vi "Parse Parameter.vi"(6 "error text in":string, 7 "direction":T1, 8 "error in":errorcluster, 11 "node in":refnum<k20>) -> (0 "error out":errorcluster, 3 "parametesrs":T2[](array[typedef]))   [LabVIEW 2023, in "ARINC 429 Import.lvlib"]
uses:
  ARINC 429 Import.lvlib
  <vilib>/NI/NI VeriStand Encoding and Decoding/Encoding.ctl
  Read Tag Element (String).vi
  Read Tag Element (DBL).vi
  Read Tag Element (I32).vi
  Shared/Parameter Definition.ctl
  Shared/VS Channel Definition for Parameter.ctl
  Read Tag Element (Boolean).vi
  Shared/Direction.ctl
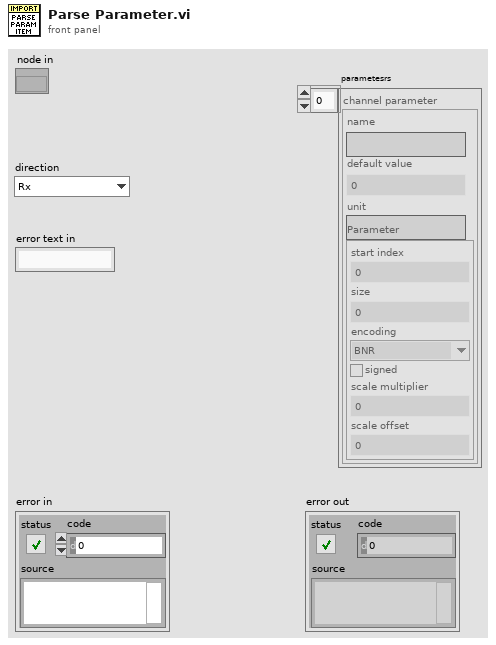
[diagram p1: front panel]
types:
  T1 = typedef "Direction.ctl" = enum16{"Rx", "Tx"}
  T2 = typedef "VS Channel Definition for Parameter.ctl" = cluster{"name":string, "default value":dbl, "unit":string, "Parameter":T3}
  T3 = typedef "Parameter Definition.ctl" = cluster{"start index":i32, "size":i32, "encoding":T4, "signed":bool, "scale multiplier":dbl, "scale offset":dbl}
  T4 = typedef "Encoding and Decoding.lvlib/Encoding.ctl" = enum16{"BNR", "BCD", "Discrete"}
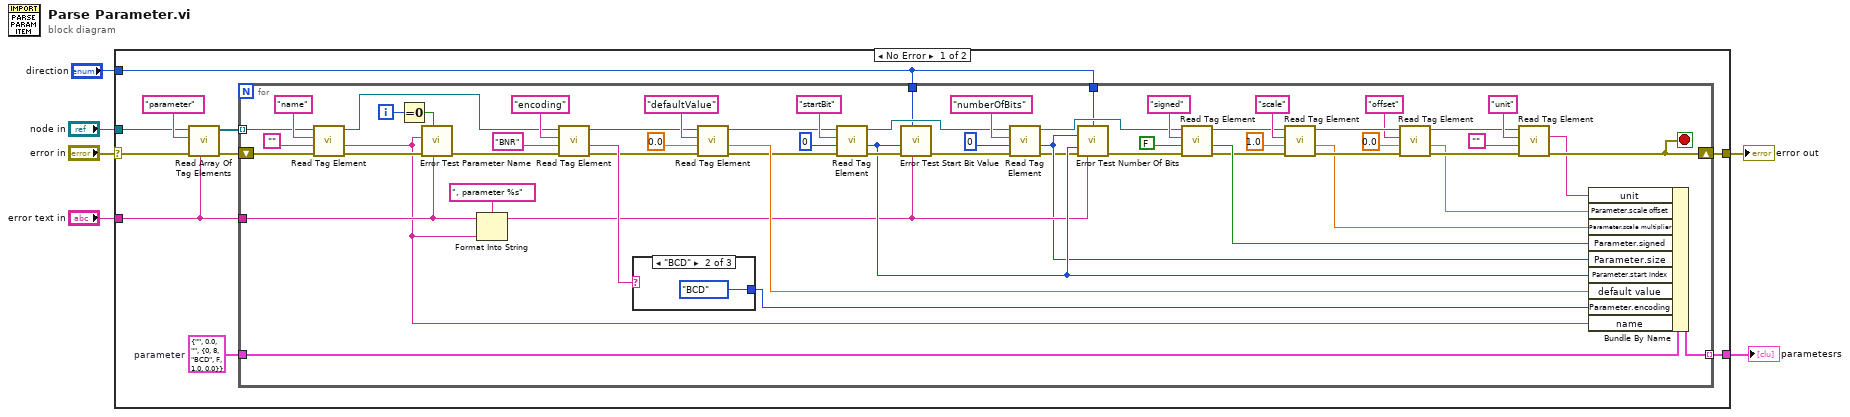
[diagram p0: block diagram]
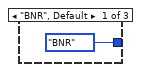
[diagram p2: hidden frame]
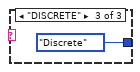
[diagram p3: hidden frame]
diagram:
  n1 = case shown="No Error" "error in" {
    selector: "error in" -> [w11 w79]
    tunnel: "node in" -> [w13 _]
    tunnel: [w12 w79] -> w5
    tunnel: "error text in" -> [w10 _]
    tunnel: [w9 _] -> w2
    tunnel: "direction" -> [w7 _]
    frame No Error {
      w8 = T2 {"name"="", "default value"=0.0, "unit"="", "Parameter"={"start index"=0, "size"=8, "encoding"=enum."BCD", "signed"=FALSE, "scale multiplier"=1.0, "scale offset"=0.0}}  # parameter
      n2 = call "Read Array Of Tag Elements.vi"("error text in"=w10, "error in"=w11, "tag name"="parameter" ("Tag Name"), "node in"=w13) -> ("error out"=w15:errorcluster, "array of elements"=w14:refnum<k20>[])  [unwired: 6 in]
      n3 = for {
        shift-right: [w38] -> w12
        shift-left: w15 -> [w73]
        tunnel: w14 -> [w41] mode=indexing
        tunnel: w10 -> [w31]
        tunnel: [w25] -> w9 mode=indexing
        tunnel: w8 -> [w24]
        tunnel: w7 -> [w23]
        tunnel: w7 -> [w20]
        i -> [w34]
        stop <- w38 stop-if-true
        n4 = call-poly "Read Tag Element.vi"("error in"=w73, "default"="", "Tag Name"="name", "node in"=w41) -> ("error out"=w36:errorcluster, "value"=w29:string, "node out"=w32:refnum<k20>)  [unwired: 5 in]
        n5 = Equal To 0?(x=w34) -> (x = 0?=w33:bool)
        n6 = call "Error Test Parameter Name.vi"("error text in"=w31, "reset (F)"=w33, "error in"=w36, "parameter name"=w29) -> ("error out"=w35:errorcluster)  [unwired: 7 in]
        n7 = Format Into String(format string=", parameter %s", initial string=w31, w29) -> (resulting string=w21:string)  [unwired: 1 in, 1 out]
        n8 = call-poly "Read Tag Element.vi"("error in"=w35, "default"="BNR", "Tag Name"="encoding", "node in"=w32) -> ("error out"=w66:errorcluster, "value"=w70:string, "node out"=w67:refnum<k20>)  [unwired: 5 in]
        n9 = case shown="\"BCD\"" w70 {
          tunnel: [Encoding."BNR" ("Encoding Type") Encoding."BCD" ("Encoding Type") Encoding."Discrete" ("Encoding Type")] -> w30
          frame "BNR", Default {
          }
          frame "BCD" {
          }
          frame "DISCRETE" {
          }
        }
        n10 = call-poly "Read Tag Element.vi"("error in"=w66, "default"=0.0, "Tag Name"="defaultValue", "node in"=w67) -> ("error out"=w58:errorcluster, "value"=w65:dbl, "node out"=w62:refnum<k20>)  [unwired: 5 in]
        n11 = call-poly "Read Tag Element.vi"("error in"=w58, "default"=0, "Tag Name"="startBit", "node in"=w62) -> ("error out"=w40:errorcluster, "value"=w22:i32, "node out"=w59:refnum<k20>)  [unwired: 5 in]
        n12 = call "Error Test Start Bit Value.vi"("error text in"=w21, "direction"=w23, "error in"=w40, "start bit"=w22) -> ("error out"=w39:errorcluster)  [unwired: 7 in]
        n13 = call-poly "Read Tag Element.vi"("error in"=w39, "default"=0, "Tag Name"="numberOfBits", "node in"=w59) -> ("error out"=w18:errorcluster, "value"=w19:i32, "node out"=w55:refnum<k20>)  [unwired: 5 in]
        n14 = call "Error Test Number Of Bits.vi"("direction"=w20, "number of bits"=w19, "start bit"=w22, "error in"=w18, "error text in"=w21) -> ("error out"=w17:errorcluster)  [unwired: 10 in]
        n15 = call-poly "Read Tag Element.vi"("error in"=w17, "default"=FALSE, "Tag Name"="signed", "node in"=w55) -> ("error out"=w46:errorcluster, "value"=w54:bool, "node out"=w47:refnum<k20>)  [unwired: 5 in]
        n16 = call-poly "Read Tag Element.vi"("error in"=w46, "default"=1.0, "Tag Name"="scale", "node in"=w47) -> ("error out"=w53:errorcluster, "value"=w26:dbl, "node out"=w52:refnum<k20>)  [unwired: 5 in]
        n17 = call-poly "Read Tag Element.vi"("error in"=w53, "default"=0.0, "Tag Name"="offset", "node in"=w52) -> ("error out"=w42:errorcluster, "value"=w27:dbl, "node out"=w43:refnum<k20>)  [unwired: 5 in]
        n18 = call-poly "Read Tag Element.vi"("error in"=w42, "default"="", "Tag Name"="unit", "node in"=w43) -> ("error out"=w38:errorcluster, "value"=w28:string)  [unwired: 5 in, 1 out]
        n19 = Bundle By Name(cluster=w24, "unit"=w28, "Parameter.scale offset"=w27, "Parameter.scale multiplier"=w26, "Parameter.signed"=w54, "Parameter.size"=w19, "Parameter.start index"=w22, "default value"=w65, "Parameter.encoding"=w30, "name"=w29) -> (w25:T2)
      }
    }
    frame Error {
    }
  }
  "parametesrs" <- w2
  "error out" <- w5
